vi "ADIS16470 Scale Data.vi"(3 "TimeStamp":u32, 5 "Data In":u8[](array[numeric])) -> (1 "Scaled Data Out":dbl[](array[numeric]), 2 "Sequence Number":u16)   [LabVIEW 2019]
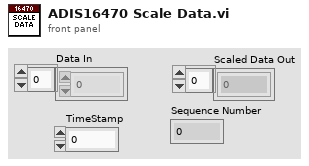
[diagram p1: front panel]
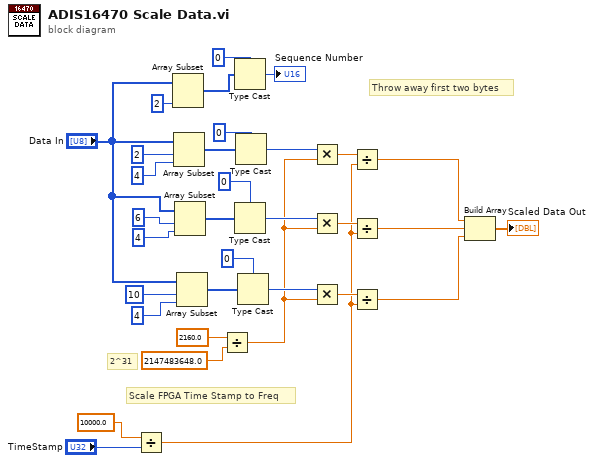
[diagram p0: block diagram]
diagram:
  # "Scale FPGA Time Stamp to Freq"
  # "2^31"
  # "Throw away first two bytes"
  n1 = Divide(x=10000.0, y="TimeStamp") -> (x/y=w6:dbl)
  n2 = Array Subset(array="Data In", length=2) -> (w2:u8[])  [unwired: 1 in]
  n3 = Array Subset(array="Data In", index=2, length=4) -> (w27:u8[])
  n4 = Array Subset(array="Data In", index=6, length=4 ("index")) -> (w25:u8[])
  n5 = Array Subset(array="Data In", index=10, length=4) -> (w26:u8[])
  n6 = Divide(x=2160.0, y=2147483648.0) -> (x/y=w15:dbl)
  n7 = Type Cast(type=u16 0, x=w2) -> (*(type *) &x=→"Sequence Number":u16)
  n8 = Type Cast(type=0, x=w25) -> (*(type *) &x=w19:i32)
  n9 = Type Cast(type=0, x=w27) -> (*(type *) &x=w21:i32)
  n10 = Type Cast(type=0, x=w26) -> (*(type *) &x=w20:i32)
  n11 = Multiply(x=w21, y=w15) -> (x*y=w14:dbl)
  n12 = Multiply(x=w19, y=w15) -> (x*y=w13:dbl)
  n13 = Multiply(x=w20, y=w15) -> (x*y=w12:dbl)
  n14 = Divide(x=w14, y=w6) -> (x/y=w9:dbl)
  n15 = Divide(x=w13, y=w6) -> (x/y=w10:dbl)
  n16 = Divide(x=w12, y=w6) -> (x/y=w11:dbl)
  n17 = Build Array(w9, w10, w11) -> (→"Scaled Data Out":dbl[])
